vi "Free Actor.vi"(8 "error in (no error)":errorcluster) -> (0 "error out":errorcluster caption="sortie d'erreur", 3 "Result":bool)   [LabVIEW 2020, in "Library Core.lvlib" / "Sequencer (Default).lvclass"]
uses:
  Sequencer (Default).lvclass
  Actor Test (Default)/Actor Test (Default).lvclass
  Sequencer (Default).lvclass/Sequencer (Default).ctl
  Commun VI/Library Commun.lvlib
panel:
  out "State_Actor":T1(ring)
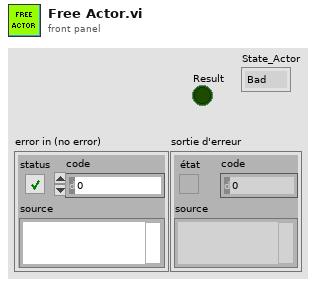
[diagram p1: front panel]
types:
  T1 = enum32{"Bad", "Idle", "Run top level", "Running"}
  T2 = enum16{"Get Actor Class", "Set Actor object", "Get Actor object", "List Actor", "Init"}
  T3 = cluster{"Name":string, "Actor Test":refnum<class "Actor Test (Default).lvclass">}[]
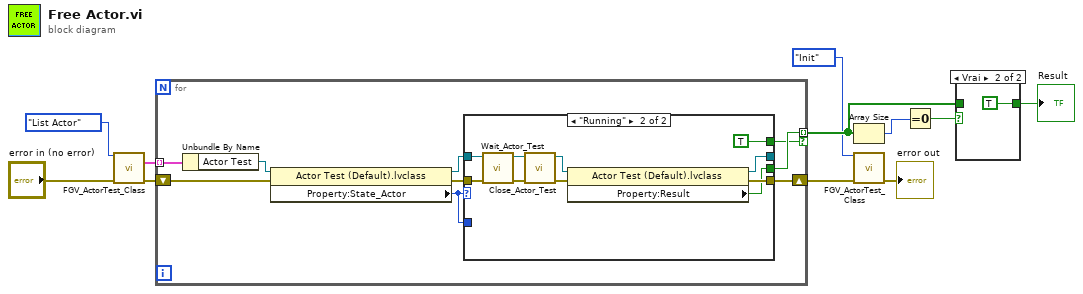
[diagram p0: block diagram]
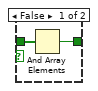
[diagram p2: hidden frame]
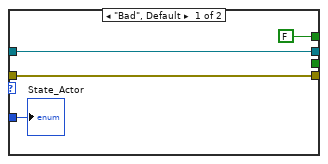
[diagram p3: hidden frame]
diagram:
  n1 = call "FGV_ActorTest_Class.vi"("Action"=T2."List Actor", "error in (no error)"="error in (no error)") -> ("List Test"=w11:T3, "error out"=w2:errorcluster)  [unwired: 10 in, 2 out]
  n2 = for {
    tunnel: w11 -> [w20] mode=indexing
    shift-right: [w13] -> w3
    shift-left: w2 -> [w18]
    tunnel: [w15] -> w6 mode=indexing if=w14
    n3 = Unbundle By Name(w20) -> ("Actor Test"=w19:refnum<class "Actor Test (Default).lvclass">)
    n4 = property class="Actor Test (Default).lvclass"(reference=w19, error in=w18) -> (reference out=w16:refnum<class "Actor Test (Default).lvclass">, error out=w17:errorcluster, "Property:State_Actor"=w12:T1)
    n5 = case shown="\"Running\"" w12 {
      tunnel: w16 -> [w24 w26]
      tunnel: w17 -> [w23 w33]
      tunnel: [w24 w31] -> _
      tunnel: [w23 w32] -> w13
      tunnel: [_ w30] -> w15
      tunnel: [FALSE TRUE] -> w14
      tunnel: w12 -> [w21 _]
      frame "Bad", Default {
        "State_Actor" <- w21
      }
      frame "Running" {
        n6 = call-dynamic "Wait_Actor_Test.vi"("error in (no error)"=w33, "Test (Default) en entrée"=w26) -> ("error out"=w28:errorcluster, "Test (Default) en sortie"=w34:refnum<class "Actor Test (Default).lvclass">)  [unwired: 8 in]
        n7 = call-dynamic "Close_Actor_Test.vi"("error in (no error)"=w28, "Test (Default) en entrée"=w34) -> ("error out"=w25:errorcluster, "Test (Default) en sortie"=w27:refnum<class "Actor Test (Default).lvclass">)  [unwired: 8 in]
        n8 = property class="Actor Test (Default).lvclass"(reference=w27, error in=w25) -> (reference out=w31:refnum<class "Actor Test (Default).lvclass">, error out=w32:errorcluster, "Property:Result"=w30:bool)
      }
    }
  }
  n9 = Array Size(array=w6) -> (size(s)=w5:i32)
  n10 = call "FGV_ActorTest_Class.vi"("Action"=T2."Init", "error in (no error)"=w3) -> ("error out"=→"error out":errorcluster)  [unwired: 10 in, 3 out]
  n11 = Equal To 0?(x=w5) -> (x = 0?=w4:bool)
  n12 = case shown="Vrai" w4 {
    tunnel: [w36 TRUE] -> w7
    tunnel: w6 -> [w35 _]
    frame False {
      n13 = And Array Elements(Boolean array=w35) -> (logical AND=w36:bool)
    }
    frame True {
    }
  }
  "Result" <- w7
